vi "Read Sampling Rate Bits.vi"(8 "error in (no error)":errorcluster, 11 "LINX-ADS1X15 in":refnum<class "LINX-ADS1X15.lvclass">) -> (0 "error out":errorcluster, 2 "Sampling Rate Bits":u16, 3 "LINX-ADS1X15 out":refnum<class "LINX-ADS1X15.lvclass">)   [LabVIEW 2020, in "LINX-ADS1X15.lvclass"]
uses:
  LINX-ADS1X15.lvclass
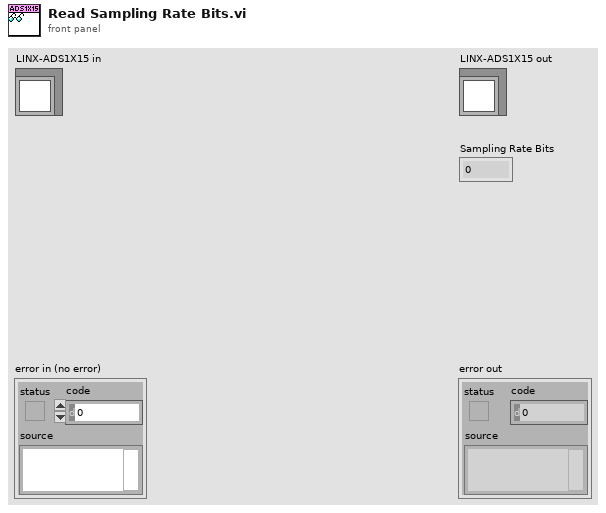
[diagram p1: front panel]
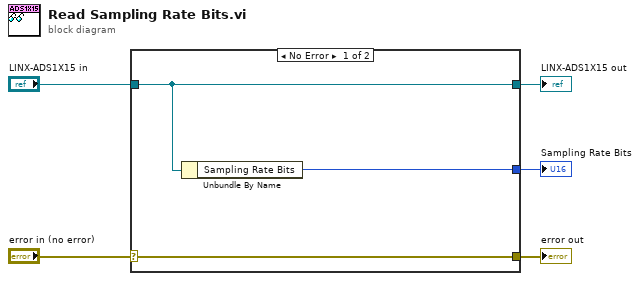
[diagram p0: block diagram]
diagram:
  n1 = case shown="No Error" "error in (no error)" {
    selector: "error in (no error)" -> [w8 w9]
    tunnel: [w8 w9] -> w4
    tunnel: [w7 w10] -> w2
    tunnel: "LINX-ADS1X15 in" -> [w7 w10]
    tunnel: [w6 _] -> w1
    frame No Error {
      n2 = Unbundle By Name(w7) -> ("Sampling Rate Bits"=w6:u16)
    }
    frame Error {
    }
  }
  "error out" <- w4
  "LINX-ADS1X15 out" <- w2
  "Sampling Rate Bits" <- w1
